vi "Sequence_Message_initial_line.vi"(0 "reference":refnum<vi>, 1 "error check?":bool, 3 "error in (no error)":errorcluster) -> (7 "Number of begin":u16, 8 "Run?":bool, 10 "error out":errorcluster)   [LabVIEW 2025]
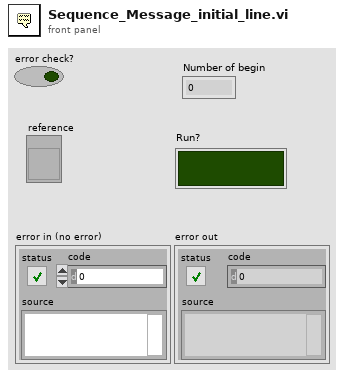
[diagram p1: front panel]
types:
  T1 = enum16{"Left Button", "Center Button", "Right Button", "Window Close"}
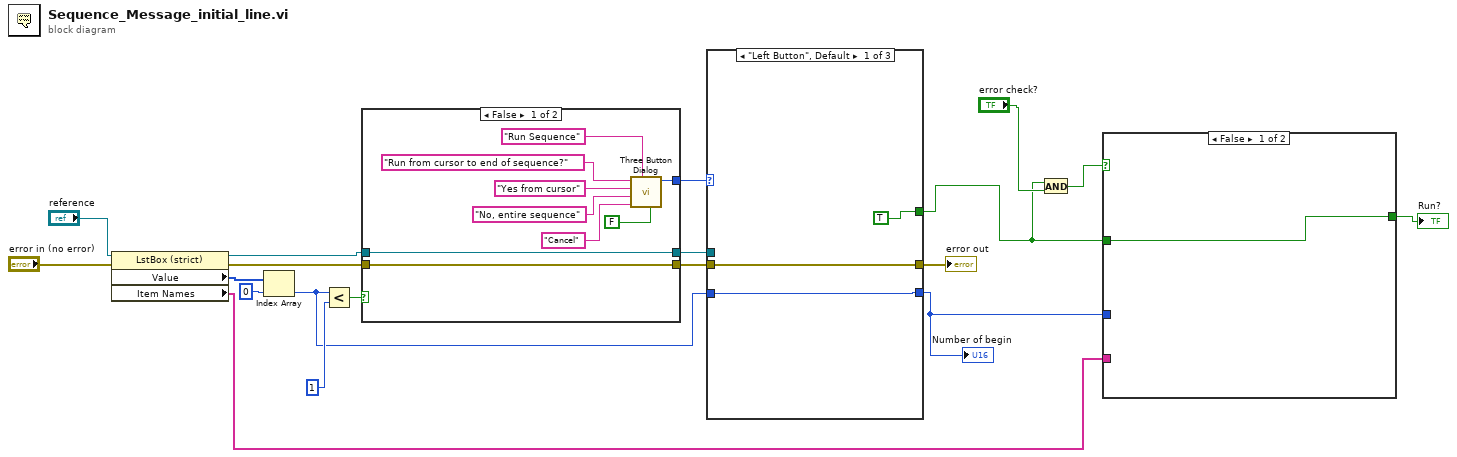
[diagram p0: block diagram]
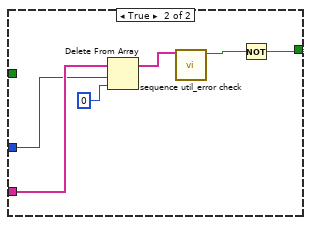
[diagram p2: hidden frame]
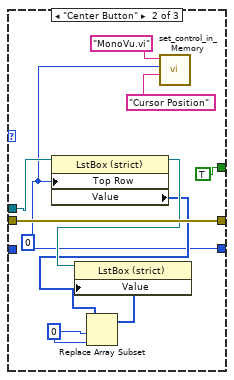
[diagram p3: hidden frame]
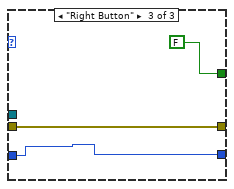
[diagram p4: hidden frame]
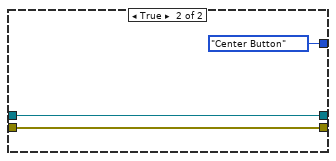
[diagram p5: hidden frame]
diagram:
  n1 = property on="Property Node" class="LstBox (strict)"(reference="reference", error in="error in (no error)") -> (reference out=w11:refnum<vi>, error out=w12:errorcluster, "Value"=w8:i32[], "Item Names"=w6:string[])
  n2 = Index Array(array=w8, index=0) -> (element=w4:i32)
  n3 = Less?(x=w4, y=1) -> (x < y?=w19:bool)
  n4 = case shown="False" w19 {
    tunnel: [w22 T1."Center Button" ("Which Button?")] -> w18
    tunnel: w12 -> [w21 w30]
    tunnel: [w21 w30] -> w17
    tunnel: w11 -> [w20 w29]
    tunnel: [w20 w29] -> w16
    frame False {
      n5 = call <vilib>:"Three Button Dialog.vi"("Allow user to close window? (TRUE)"=FALSE, "Window Title (\"\")"="Run Sequence" ("message"), "Right Button Text (\"Cancel\")"="Cancel" ("Right Button Text (\"Cancel\")"), "Center Button Text (\"No\")"="No, entire sequence" ("Left Button Text (\"Yes\")"), "Left Button Text (\"Yes\")"="Yes from cursor" ("Left Button Text (\"Yes\")"), "message"="Run from cursor to end of sequence?" ("Center Button Text (\"No\")")) -> ("Which Button?"=w22:T1)  [unwired: 5 in]
    }
    frame True {
    }
  }
  n6 = case shown="\"Left Button\", Default" w18 {
    tunnel: w17 -> [w32 w44 w47]
    tunnel: w16 -> [_ w42 _]
    tunnel: [TRUE TRUE FALSE] -> w1
    tunnel: [w32 w44 w47] -> w15
    tunnel: [w33 w35 w46] -> w5
    tunnel: w4 -> [w33 _ w46]
    frame "Left Button", Default {
    }
    frame "Center Button" {
      w39 = 0 ("index")
      w35 = u16 0 ("Number of begin")
      n7 = property on="Property Node" class="LstBox (strict)"(reference=w42, "Top Row"=w35) -> (reference out=w41:refnum<vi>, "Value"=w40:i32[])  [unwired: 1 in, 1 out]
      n8 = Replace Array Subset(array=w40, new element=w39, index=w39) -> (w38:i32[])
      n9 = property on="Property Node" class="LstBox (strict)"(reference=w41, "Value"=w38) -> ()  [unwired: 1 in, 2 out]
      n10 = call "set_control_in_Memory.vi"("Control Name"="Cursor Position", "Value"=w35, "VI Name"="MonoVu.vi") -> ()  [unwired: 2 in, 1 out]
    }
    frame "Right Button" {
    }
  }
  "error out" <- w15
  "Number of begin" <- w5
  n11 = And(x=w1, y="error check?") -> (x .and. y?=w2:bool)
  n12 = case shown="False" w2 {
    tunnel: w1 -> [w48 _]
    tunnel: [w48 w54] -> w7
    tunnel: w6 -> [_ w53]
    tunnel: w5 -> [_ w52]
    frame False {
    }
    frame True {
      n13 = Delete From Array(array=w53, length=w52, index=0) -> (array with subset deleted=w50:string[])  [unwired: 1 out]
      n14 = call "sequence util_error check.vi"("Item Names IN"=w50) -> ("error"=w49:bool)  [unwired: 8 in, 1 out]
      n15 = Not(x=w49) -> (.not. x?=w54:bool)
    }
  }
  "Run?" <- w7
